vi "symlimit.vi"(1 "Limit":i16, 2 "Input Sig":i16) -> (0 "Output Sig":i16)   [LabVIEW 2010, in "Wall Follower.lvrbt"]
uses:
  Wall Follower.lvrbt
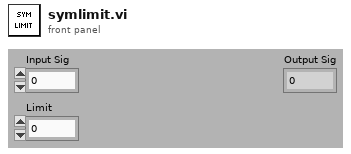
[diagram p1: front panel]
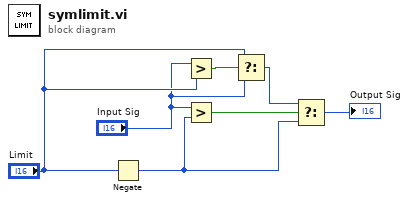
[diagram p0: block diagram]
diagram:
  n1 = Negate(x="Limit") -> (-x=w3:i16)
  n2 = Greater?(x="Input Sig", y="Limit") -> (0:w7:bool)
  n3 = Greater?(x="Input Sig", y=w3) -> (0:w4:bool)
  n4 = Select(t="Limit", s=w7, f="Input Sig") -> (s? t:f=w2:i16)
  n5 = Select(t=w2, s=w4, f=w3) -> (s? t:f=→"Output Sig":i16)
